vi "Rename.vi"() -> ()   [LabVIEW 2021]
uses:
  <vilib>/Utility/EditLVLibs/Edit LVLibs.lvlib
  _Rename/_Rename.lvlib
panel:
  in  "Rename":bool
  in  "Rename":string
  in  "Msgs":string(combo)
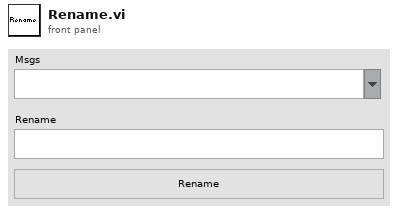
[diagram p1: front panel]
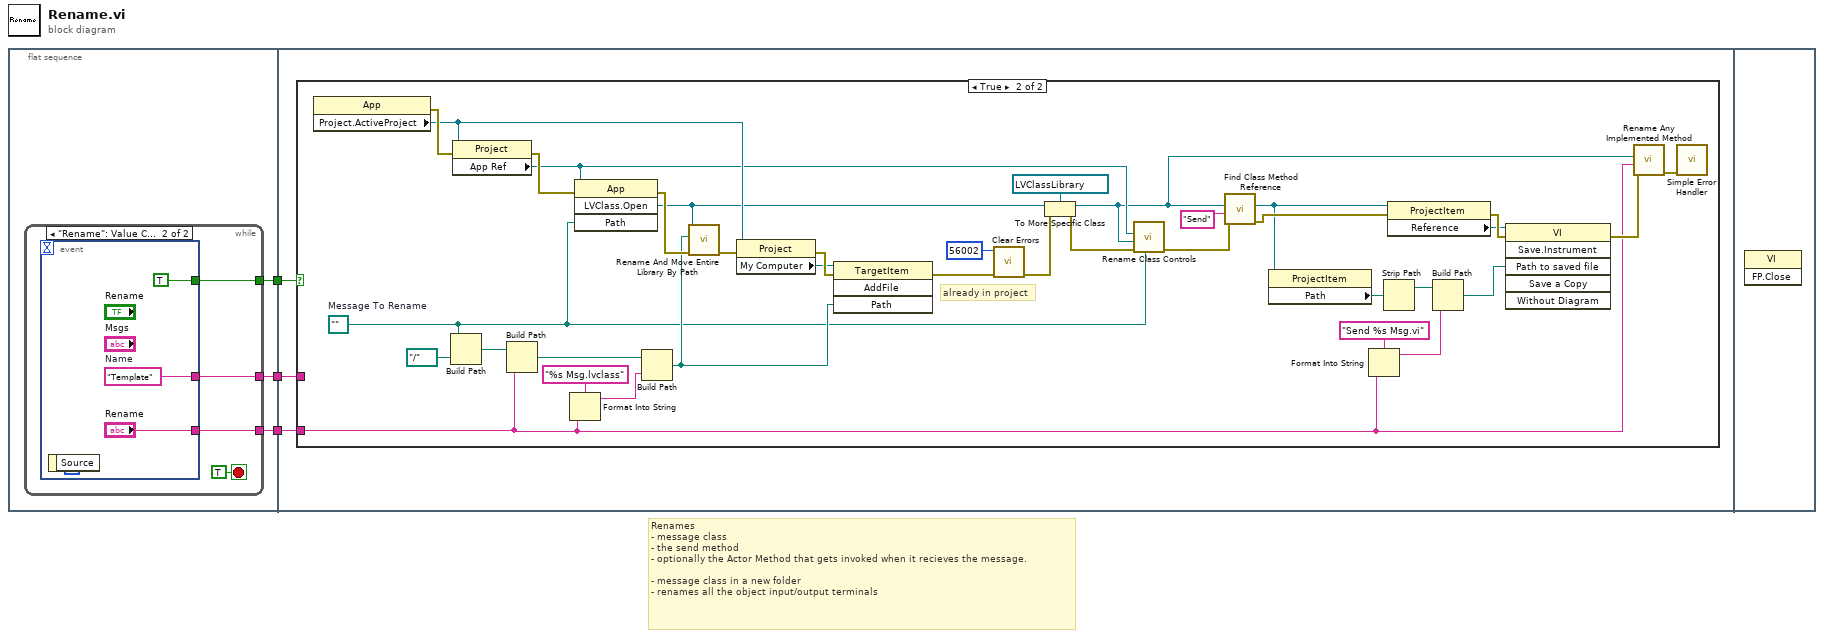
[diagram p0: block diagram]
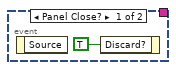
[diagram p2: hidden frame]
diagram:
  # "Renames\n- message class\n- the send method\n- optionally the Actor Method that gets invoked when it recieves the message.\n\n- message class in a new folder\n- renames all the object input/output terminals"
  n1 = flat-sequence {
    tunnel: [w6] -> w3
    tunnel: [w5] -> w2
    tunnel: [w4] -> w1
    tunnel: w3 -> [w17]
    tunnel: w2 -> [w16]
    tunnel: w1 -> [w15]
    frame #0 {
      n2 = while {
        tunnel: [w10] -> w6
        tunnel: [w9] -> w5
        tunnel: [w7] -> w4
        stop <- TRUE stop-if-true
        n3 = event shown="[1] \"Rename\": Value Change" {
          selector: _ -> [_ _]
          dyn-events: _ -> [_ _]
          timeout: _ -> [_ _]
          tunnel: [_ TRUE ("Rename 2")] -> w10
          tunnel: [_ "Rename"] -> w9
          tunnel: [_ w12] -> w7
          event Panel Close? {
            n4 = event-data() -> ()  [unwired: 1 in, 1 out]
            n5 = event-data("Discard?"=TRUE) -> ()  [unwired: 1 in, 1 out]
          }
          event "Rename": Value Change {
            w12 = "Template"  # Name
            n6 = event-data() -> ()  [unwired: 1 in, 1 out]
          }
        }
      }
    }
    frame #1 {
      n7 = case shown="True" w17 {
        tunnel: w16 -> [_ w19]
        tunnel: w15 -> [_ _]
        frame False {
        }
        frame True {
          w30 = path ""  # Message To Rename
          # "already in project"
          n8 = property class="App"() -> (error out=w50:errorcluster, "Project.ActiveProject"=w35:refnum<vi>)  [unwired: 2 in, 1 out]
          n9 = Build Path(base path=w30, name or relative path=path "../..") -> (appended path=w44:path)
          n10 = property class="Project"(reference=w35, error in=w50) -> (error out=w46:errorcluster, "App Ref"=w33:refnum<vi>)  [unwired: 1 out]
          n11 = Build Path(base path=w44, name or relative path=w19) -> (appended path=w43:path)
          n12 = Format Into String(format string="%s Msg.lvclass", w19) -> (resulting string=w20:string)  [unwired: 2 in, 1 out]
          n13 = invoke class="App" method="LVClass.Open"(reference=w33, error in=w46, "Path"=w30) -> (error out=w49:errorcluster, "LVClass.Open"=w18:refnum<vi>)  [unwired: 1 in, 2 out]
          n14 = Build Path(base path=w43, name or relative path=w20) -> (appended path=w42:path)
          n15 = call <vilib>:"Rename And Move Entire Library By Path.vi"("error in (no error)"=w49, "New library path"=w42, "Library ref in"=w18) -> ("error out"=w34:errorcluster)  [unwired: 7 in, 1 out]
          n16 = property class="Project"(reference=w35, error in=w34) -> (error out=w53:errorcluster, "My Computer"=w36:refnum<vi>)  [unwired: 1 out]
          n17 = invoke class="TargetItem" method="AddFile"(reference=w36, error in=w53, "Path"=w42) -> (error out=w51:errorcluster)  [unwired: 1 in, 3 out]
          n18 = call <vilib>:"Clear Errors.vi"("error in (no error)"=w51, "specific error code to clear (0: all)"=56002) -> ("error out"=w48:errorcluster)  [unwired: 4 in, 1 out]
          n19 = To More Specific Class(target class=refnum<vi> refnum ("Class in"), reference=w18, error in=w48) -> (specific class reference=w26:refnum<vi>, error out=w47:errorcluster)
          n20 = call "Rename Class Controls.vi"("Old Class"=w30, "error in"=w47, "Class to Rename"=w26, "App Ref"=w33) -> ("error out"=w27:errorcluster)  [unwired: 7 in]
          n21 = call "Find Class Method Reference.vi"("error in"=w27, "Method Name"="Send" ("regular expression"), "Class Reference"=w26) -> ("error out"=w25:errorcluster, "Method Reference"=w24:refnum<vi>)  [unwired: 7 in]
          n22 = property class="ProjectItem"(reference=w24) -> ("Path"=w29:path)  [unwired: 1 in, 2 out]
          n23 = Format Into String(format string="Send %s Msg.vi", w19) -> (resulting string=w22:string)  [unwired: 2 in, 1 out]
          n24 = Strip Path(path=w29) -> (stripped path=w41:path)  [unwired: 1 out]
          n25 = property class="ProjectItem"(reference=w24, error in=w25) -> (error out=w52:errorcluster, "Reference"=w40:refnum<vi>)  [unwired: 1 out]
          n26 = Build Path(base path=w41, name or relative path=w22) -> (appended path=w39:path)
          n27 = invoke class="VI" method="Save.Instrument"(reference=w40, error in=w52, "Path to saved file"=w39) -> (error out=w31:errorcluster)  [unwired: 3 in, 5 out]
          n28 = call "Rename Any Implemented Method.vi"("error in"=w31, "Name"=w19, "Class To Rename"=w26) -> ("error out"=w32:errorcluster)  [unwired: 8 in]
          n29 = call <vilib>:"Simple Error Handler.vi"("error in (no error)"=w32) -> ()  [unwired: 4 in, 5 out]
        }
      }
    }
    frame #2 {
      n30 = invoke class="VI" method="FP.Close"() -> ()  [unwired: 3 in, 3 out]
    }
  }
